vi "Test Cryogens.vi"(8 "error in (no error)":errorcluster, 11 "Instrument.Cryostat in":refnum<class "Instrument.Cryostat.lvclass">) -> (0 "error out":errorcluster, 3 "Instrument.Cryostat out":refnum<class "Instrument.Cryostat.lvclass">)   [LabVIEW 2016]
uses:
  lvsrc/Instrument Types/Cryostat/Instrument.Cryostat.lvclass
  <vilib>/addons/_JKI Toolkits/Caraya/classes/Assert/Assert.lvclass
  <vilib>/addons/_JKI Toolkits/Caraya/classes/Test/Test.lvclass
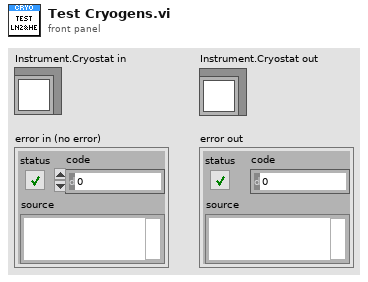
[diagram p1: front panel]
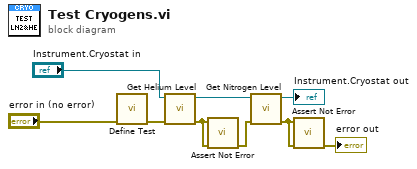
[diagram p0: block diagram]
diagram:
  n1 = call <vilib>:"Define Test.vi"("error in (no error)"="error in (no error)") -> ("error out"=w1:errorcluster)  [unwired: 10 in]
  n2 = call-dynamic "Get Helium Level.vi"("error in (no error)"=w1, "Instrument.Cryostat in"="Instrument.Cryostat in") -> ("error out"=w6:errorcluster, "Instrument.Cryostat out"=w5:refnum<class "Instrument.Cryostat.lvclass">)  [unwired: 7 in, 1 out]
  n3 = call <vilib>:"Assert Not Error.vi"("error in (no error)"=w6, "Not Error?"=w6) -> ("error out"=w7:errorcluster)  [unwired: 9 in]
  n4 = call-dynamic "Get Nitrogen Level.vi"("error in (no error)"=w7, "Instrument.Cryostat in"=w5) -> ("error out"=w8:errorcluster, "Instrument.Cryostat out"=→"Instrument.Cryostat out":refnum<class "Instrument.Cryostat.lvclass">)  [unwired: 7 in, 1 out]
  n5 = call <vilib>:"Assert Not Error.vi"("error in (no error)"=w8, "Not Error?"=w8) -> ("error out"=→"error out":errorcluster)  [unwired: 9 in]
